vi "Write anotherNumber.vi"(8 "error in (no error)":errorcluster, 10 "anotherNumber":dbl, 11 "Test2 in":refnum<class "Class2.lvclass">) -> (0 "error out":errorcluster, 3 "Test2 out":refnum<class "Class2.lvclass">)   [LabVIEW 2020, in "Class2.lvclass"]
doc: "GCraftsman JSON Object Serialization Toolkit\nwww.GCraftsman.com\nCopyright (c) 2017, GCraftsman"
uses:
  Class2.lvclass
  Class2.lvclass/Class2.ctl
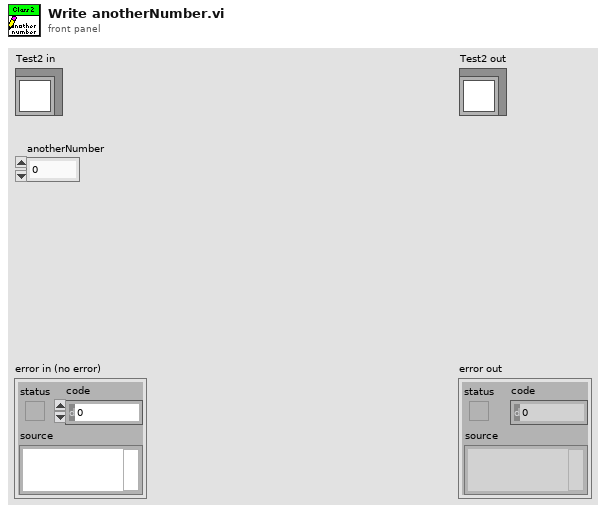
[diagram p1: front panel]
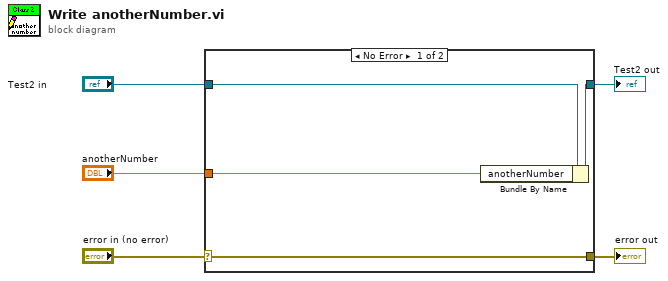
[diagram p0: block diagram]
diagram:
  n1 = case shown="No Error" "error in (no error)" {
    selector: "error in (no error)" -> [w9 w10]
    tunnel: [w9 w10] -> w4
    tunnel: [w7 w11] -> w2
    tunnel: "Test2 in" -> [w8 w11]
    tunnel: "anotherNumber" -> [w6 _]
    frame No Error {
      n2 = Bundle By Name(cluster=w8, "anotherNumber"=w6) -> (w7:refnum<class "Class2.lvclass">)
    }
    frame Error {
    }
  }
  "error out" <- w4
  "Test2 out" <- w2
